vi "Strip Cluster (Variant).vi"(7 "Prefix Name":string, 8 "error in (no error)":errorcluster, 9 "Values in":variant[](array[variant]), 10 "Key in":string[](array[string]), 11 "Cluster Refnum":refnum<vi>) -> (0 "error out":errorcluster, 1 "Values":variant[](array[variant]), 2 "Keys":string[](array[string]), 3 "Cluster Refnum (Dup)":refnum<vi>)   [LabVIEW 2017]
doc: "Wire any cluster control reference to this VI. The VI will generate keys and values for each element of the cluster. The operation is recursive, so keys will be generated for array and cluster elements as well. The key and value inputs are required to support recursion, but may be used to chain the outputs of multiple strip operations over several clusters.\n\nSupported data types, as of 12/20/06:\nBoolean (TRUE if value is <> 0 or <> \"FALSE\")\nPath\nDouble\nString\nEnumerated Type (value can be an integer or enum string)\nTime stamp (value saved as a double)\nArray (recursive)\nCluster (recursive)\nShared Variable Reference\nRing Control (value can be an integer or string)\nVISA resource name\nCombo Box (value can be the string or combo box value)\n\nKey format:\n<prefix>.<control name_1>[.M.<control name_2>]...[.<control name_N>]\n\nIf the <prefix> input is an empty string, the label of the input cluster will be used instead.\n\n<control name> is the name of a control in the cluster. The control may be any supported type, including arrays and clusters.\n\n<control name_N>.n.<control name_N+1> is the Mth element of the <control name_N> array, where the array element is named <control name_N+1>. The array element name is not optional."
panel:
  in  "Strip Cluster":refnum<vi>
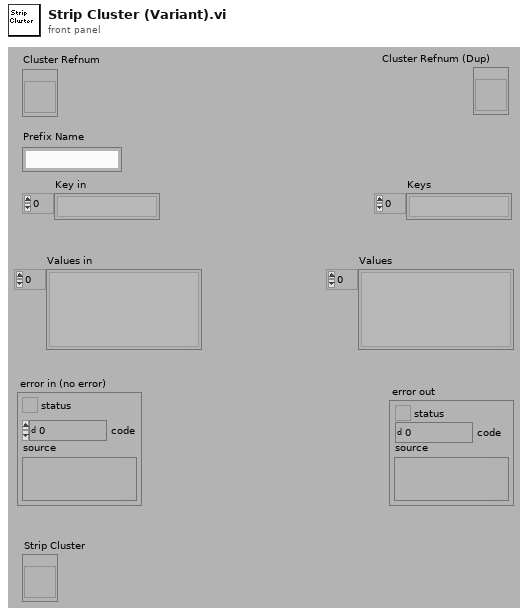
[diagram p1: front panel]
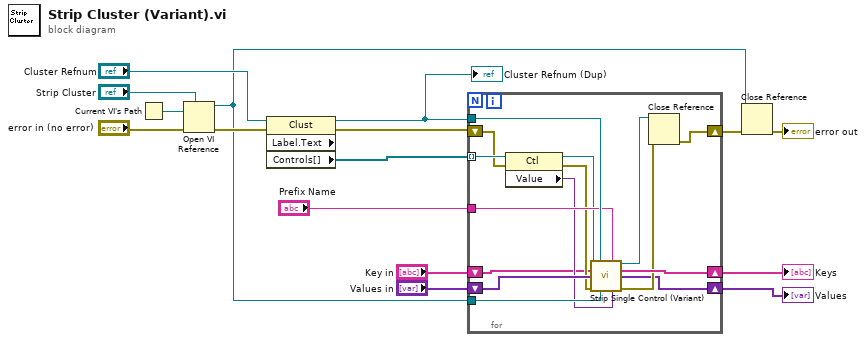
[diagram p0: block diagram]
diagram:
  n1 = Current VI's Path() -> (path=w13:path)
  n2 = Open VI Reference(type specifier VI Refnum (for type only)="Strip Cluster", vi path=w13, error in (no error)="error in (no error)") -> (vi reference=w3:refnum<vi>, error out=w11:errorcluster)  [unwired: 3 in]
  n3 = property class="Clust" props=["Label", "Text", "Controls[]"](reference="Cluster Refnum", error in=w11) -> (reference out=w9:refnum<vi>, error out=w16:errorcluster, "Controls[]"=w15:refnum<vi>[])  [unwired: 1 out]
  "Cluster Refnum (Dup)" <- w9
  n4 = for {
    tunnel: w15 -> [w26] mode=indexing
    shift-right: [w19] -> w4
    shift-left: w16 -> [w23]
    tunnel: w3 -> [w31]
    tunnel: w9 -> [w30]
    shift-right: [w17] -> w5
    shift-left: "Values in" -> [w29]
    shift-right: [w28] -> w6
    shift-left: "Key in" -> [w18]
    tunnel: "Prefix Name" -> [w27]
    n5 = property class="Ctl"(reference=w26, error in=w23) -> (reference out=w25:refnum<vi>, error out=w22:errorcluster, "Value"=w24:variant)
    n6 = call "Strip Single Control (Variant).vi"("Ctl Refnum"=w25, "Cluster Refnum"=w30, "Label.Text"=w27, "Keys in"=w18, "Values in"=w29, "error in (no error)"=w22, "Strip Cluster"=w31, "Value"=w24) -> ("Ctl Refnum"=w21:refnum<vi>, "Keys out"=w28:string[], "Values out"=w17:variant[], "error out"=w20:errorcluster)  [unwired: 4 in]
    n7 = Close Reference(reference=w21, error in (no error)=w20) -> (error out=w19:errorcluster)
  }
  "Keys" <- w6
  "Values" <- w5
  n8 = Close Reference(reference=w3, error in (no error)=w4) -> (error out=→"error out":errorcluster)
